vi "Run Service.vi"() -> ()   [LabVIEW 2024, in "Service Template.lvlib"]
uses:
  Service Template.lvlib
  gRPC lv Support/grpc-lvsupport/grpc-lvsupport.lvlib
  gRPC lv Servicer/Servicer/Servicer.lvclass
  gRPC lv Servicer/ServiceBase/ServiceBase.lvclass
panel:
  in  "Async [T] / Sync [F]":bool
  out "Listening Port":i32
  in  "Stop":bool
  in  "Server Address":string="localhost:50051"
  in  "Server Certificate File (.crt)":path
  in  "Server Key File (.key)":path
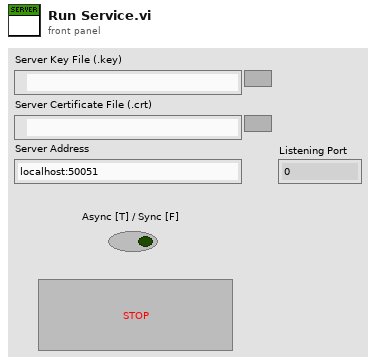
[diagram p1: front panel]
types:
  T1 = typedef "grpc-lvsupport.lvlib/grpcId.ctl" = u64
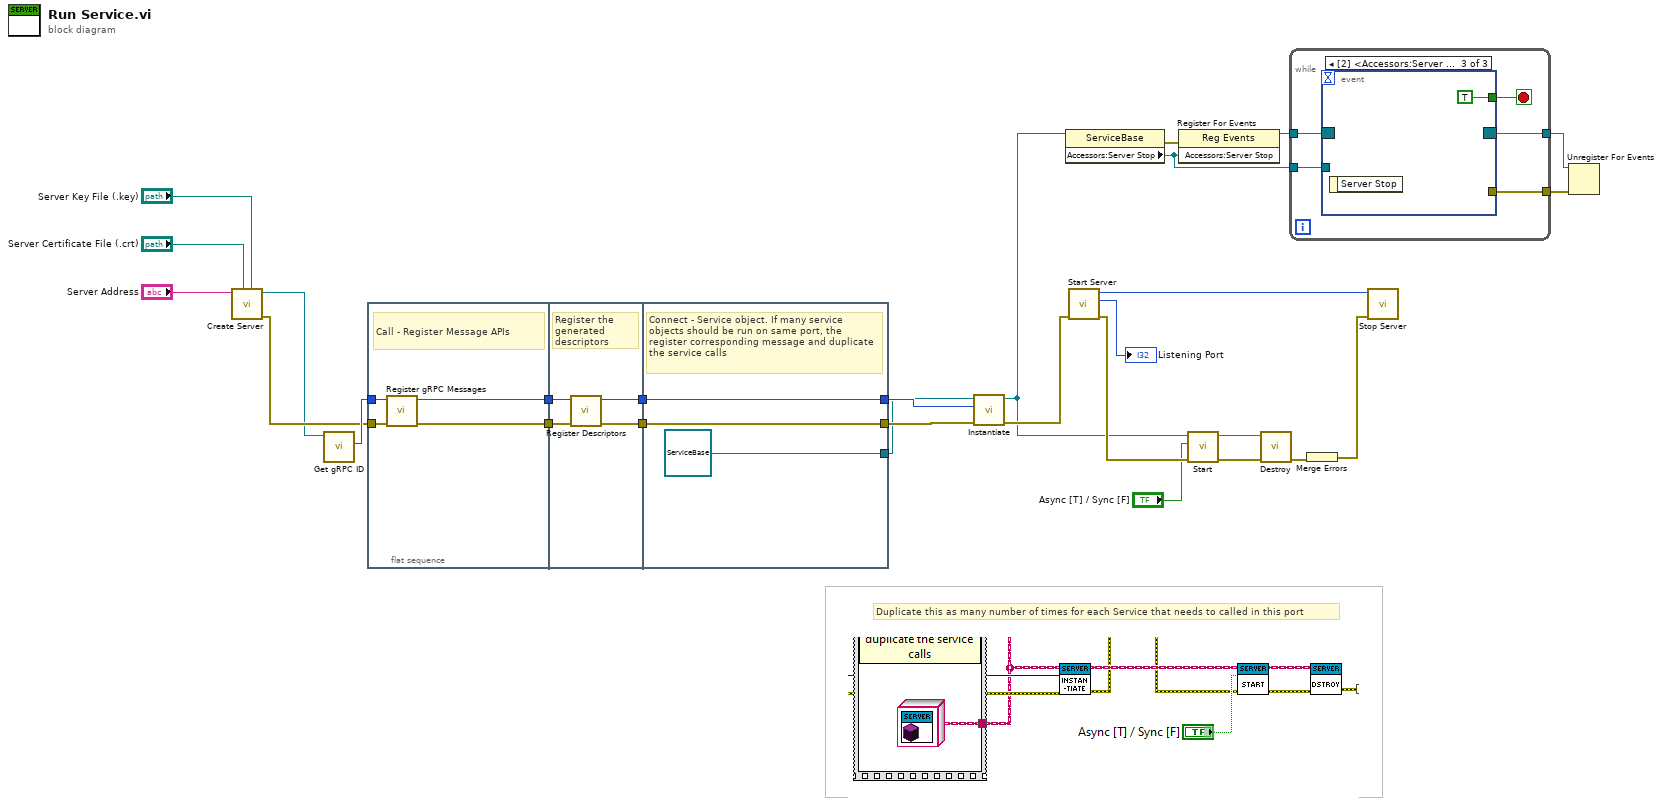
[diagram p0: block diagram]
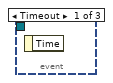
[diagram p2: hidden frame]
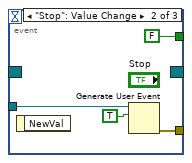
[diagram p3: hidden frame]
diagram:
  # "Duplicate this as many number of times for each Service that needs to called in this port"
  n1 = call "Create Server.vi"("Server Key File (.key)"="Server Key File (.key)", "Server Certificate File (.crt)"="Server Certificate File (.crt)", "Server Address"="Server Address") -> ("error out"=w18:errorcluster, "gRPC Server out"=w1:refnum<class "Servicer.lvclass">)  [unwired: 7 in]
  n2 = call "Get gRPC ID.vi"("OOP Server in"=w1) -> ("gRPC ID"=w19:T1)  [unwired: 9 in, 1 out]
  n3 = flat-sequence {
    tunnel: w19 -> [w30]
    tunnel: w18 -> [w32]
    tunnel: [w31] -> w9
    tunnel: [w29] -> w8
    tunnel: w9 -> [w35]
    tunnel: w8 -> [w36]
    tunnel: [w33] -> w7
    tunnel: [w34] -> w6
    tunnel: [w38] -> w16
    tunnel: [w39] -> w17
    tunnel: w7 -> [w39]
    tunnel: w6 -> [w38]
    tunnel: [refnum<class "ServiceBase.lvclass"> refnum ("gRPC-servicer.lvlib:iService.lvclass")] -> w5
    frame #0 {
      # "Call - Register Message APIs"
      n4 = call "Register gRPC Messages.vi"("error in (no error)"=w32, "gRPC ID"=w30) -> ("error out"=w31:errorcluster, "gRPC ID Out"=w29:T1)  [unwired: 8 in]
    }
    frame #1 {
      # "Register the generated descriptors"
      n5 = call "Register Descriptors.vi"("error in (no error)"=w35, "gRPC ID"=w36) -> ("error out"=w33:errorcluster, "gRPC ID Out"=w34:T1)  [unwired: 8 in]
    }
    frame #2 {
      # "Connect - Service object. If many service objects should be run on same port, the register corresponding message and duplicate the service calls"
    }
  }
  n6 = call-dynamic "Instantiate.vi"("error in"=w17, "gRPCid"=w16, "iService"=w5) -> ("error out"=w23:errorcluster, "iService"=w11:refnum<class "ServiceBase.lvclass">)  [unwired: 7 in]
  n7 = property class="ServiceBase"(reference=w11) -> (error out=w24:errorcluster, "Accessors:Server Stop"=w10:refnum<user-event>)  [unwired: 1 in, 1 out]
  n8 = call "Start Server.vi"("error in"=w23) -> ("error out"=w15:errorcluster, "Listening Port"=→"Listening Port":i32, "gRPCid server out"=w28:T1)  [unwired: 8 in]
  n9 = register-events(error in=w24, w10) -> (reference out=w27:refnum<event-registration>)  [unwired: 1 in, 1 out]
  n10 = call-dynamic "Start.vi"("error in"=w15, "ASync [T]"="Async [T] / Sync [F]", "iService in"=w11) -> ("error out"=w14:errorcluster, "iService out"=w13:refnum<class "ServiceBase.lvclass">)  [unwired: 7 in]
  n11 = call-dynamic "Destroy.vi"("error in"=w14, "SignalGeneratorService in"=w13) -> ("error out"=w22:errorcluster)  [unwired: 8 in, 1 out]
  n12 = while {
    tunnel: w27 -> [w44]
    tunnel: [w42] -> w26
    tunnel: [w40] -> w20
    tunnel: w10 -> [w41]
    stop <- w43 stop-if-true
    n13 = event shown="[2] <Accessors:Server Stop>: User Event" {
      selector: w44 -> [_ _ _]
      dyn-events: [_ _ _] -> w42
      timeout: _ -> [_ _ _]
      tunnel: [_ FALSE TRUE] -> w43
      tunnel: w41 -> [_ w47 _]
      tunnel: [_ w45 _] -> w40
      event Timeout {
        n14 = event-data() -> ()  [unwired: 1 in, 1 out]
      }
      event "Stop": Value Change {
        n15 = event-data() -> ()  [unwired: 1 in, 1 out]
        n16 = Generate User Event(user event=w47, event data cluster=TRUE ("event data")) -> (error out=w45:errorcluster)  [unwired: 2 in, 1 out]
      }
      event User Event {
        n17 = event-data() -> ()  [unwired: 1 in, 1 out]
      }
    }
  }
  n18 = Merge Errors(w22) -> (w21:errorcluster)
  n19 = call "Stop Server.vi"("error in"=w21, "gRPCid server in"=w28) -> ()  [unwired: 9 in, 1 out]
  n20 = Unregister For Events(event registration refnum=w26, error in=w20) -> ()  [unwired: 1 out]
